vi "SLM_Control_Sample.vi"() -> ()   [LabVIEW 2016]
panel:
  in  "STOP button":bool
  out "Dffraction image":picture caption="Diffraction image"
  out "LG Beam image":picture
  out "Cylindrical lense image":picture caption="Cylindrical Lens image"
  out "Axicon image":picture
  out "Target image":picture
  out "Correction image":picture
  out "CGH image":picture caption="Tiled CGH image / Target image"
  out "Fresnel Lens image":picture
  out "2nd Display(LCOS) image":picture
  in  "?":T1(tab)
  in  "CGH  ON / OFF":bool=TRUE
  in  "LCOS type":string(combo)="X15223 series"
  in  "Corection image address":path
  in  "Target image address":path
  in  "Repetition Number":u32=100
  in  "Slip":i32
  in  "Cylindrical Lens":bool=TRUE
  in  "Cylindrical Focus/mm":i32=1000
  in  "WaveFront":bool=TRUE
  in  "Fresnel Lens":bool=TRUE
  in  "LUT":bool
  in  "2π Signal Level (0-255)":u8=210
  in  "Fresnel Focus/mm":i32=1000
  in  "Wave length/nm":u32=532
  out "Wave length/nm":u32=532
  in  "Mode Select":enum32{"Row", "Column"}(radio)
  in  "Rotation degree":dbl
  in  "Axicon Lens":bool=TRUE
  in  "Top level / πrad.":dbl=4.0
  in  "LG Beam":bool=TRUE
  in  "m":u32=1
  in  "p":u32=1
  in  "Diffraction":bool=TRUE
  in  "Mode Select2":enum32{"Row", "Column"}(radio)
  in  "gradation width":u32=1
  in  "gradation number":u32=2
  in  "Flip image":i32(listbox)
  in  "Beam size / mm":dbl
  in  "Additional phase mask (2πrad. at 0-255level) 2":path
  in  "Additional phase combination mode\nComplex amplitude / Amplitude 2":bool
  in  "Save 2nd Display image button":bool
  in  "Additional phase combination mode\nComplex amplitude / Amplitude 1":bool=TRUE
  in  "Monitor mumber":i32=2
  in  "Y PixelShift":i32
  in  "X PixelShift":i32
  in  "Additional phase mask (2πrad. at 0-255level) 1":path
  # "Sample code for\nLabVIEW"
  # "Basic Setting Parameter"
  # "LCOS-SLM"
  # "If a null address was input , all 0 pattern will appear."
  # "Target image"
  # "Corection"
  # "CGH"
  # "LCOS display settings"
  # "After press the STOP button, the BMP data save dialog will open."
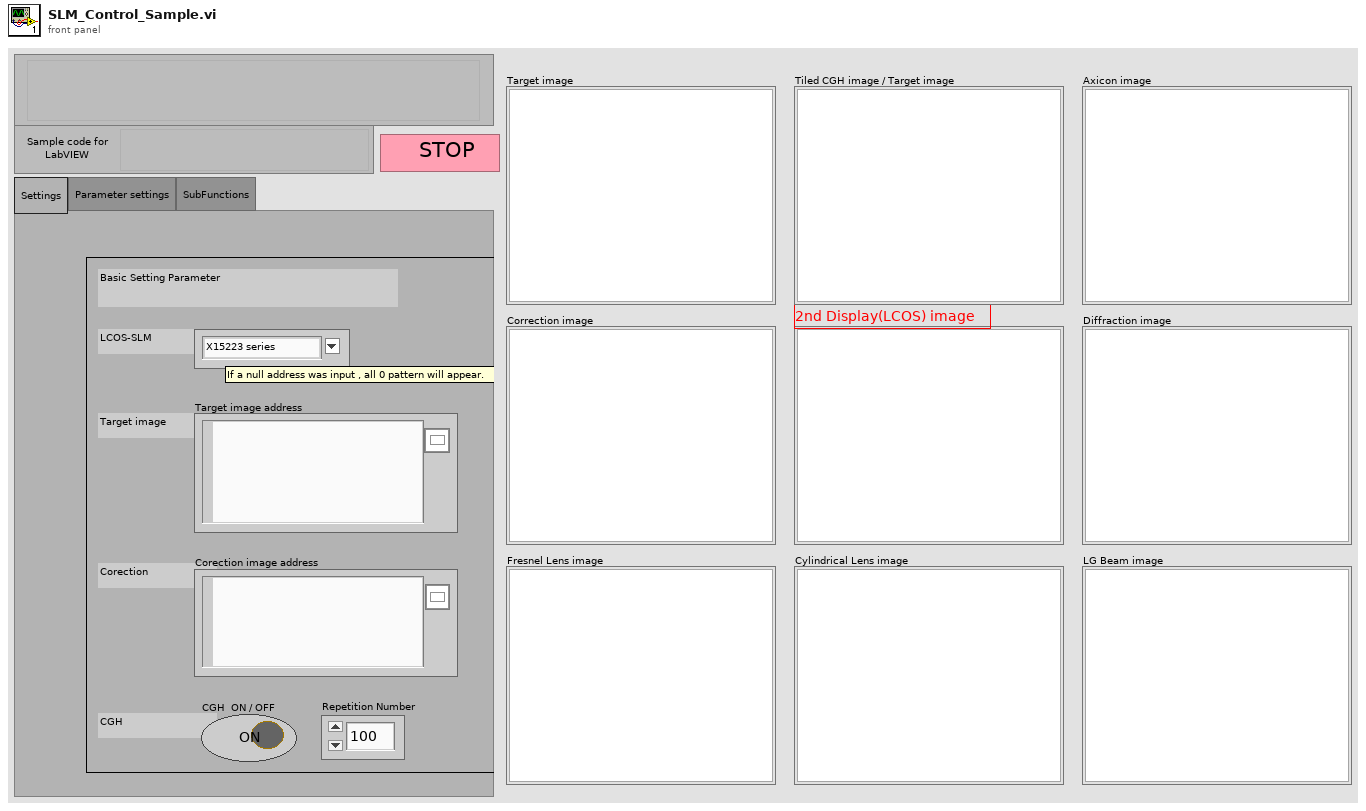
[diagram p1: front panel]
types:
  T1 = enum32{"Settings", "Parameter settings", "SubFunctions"}
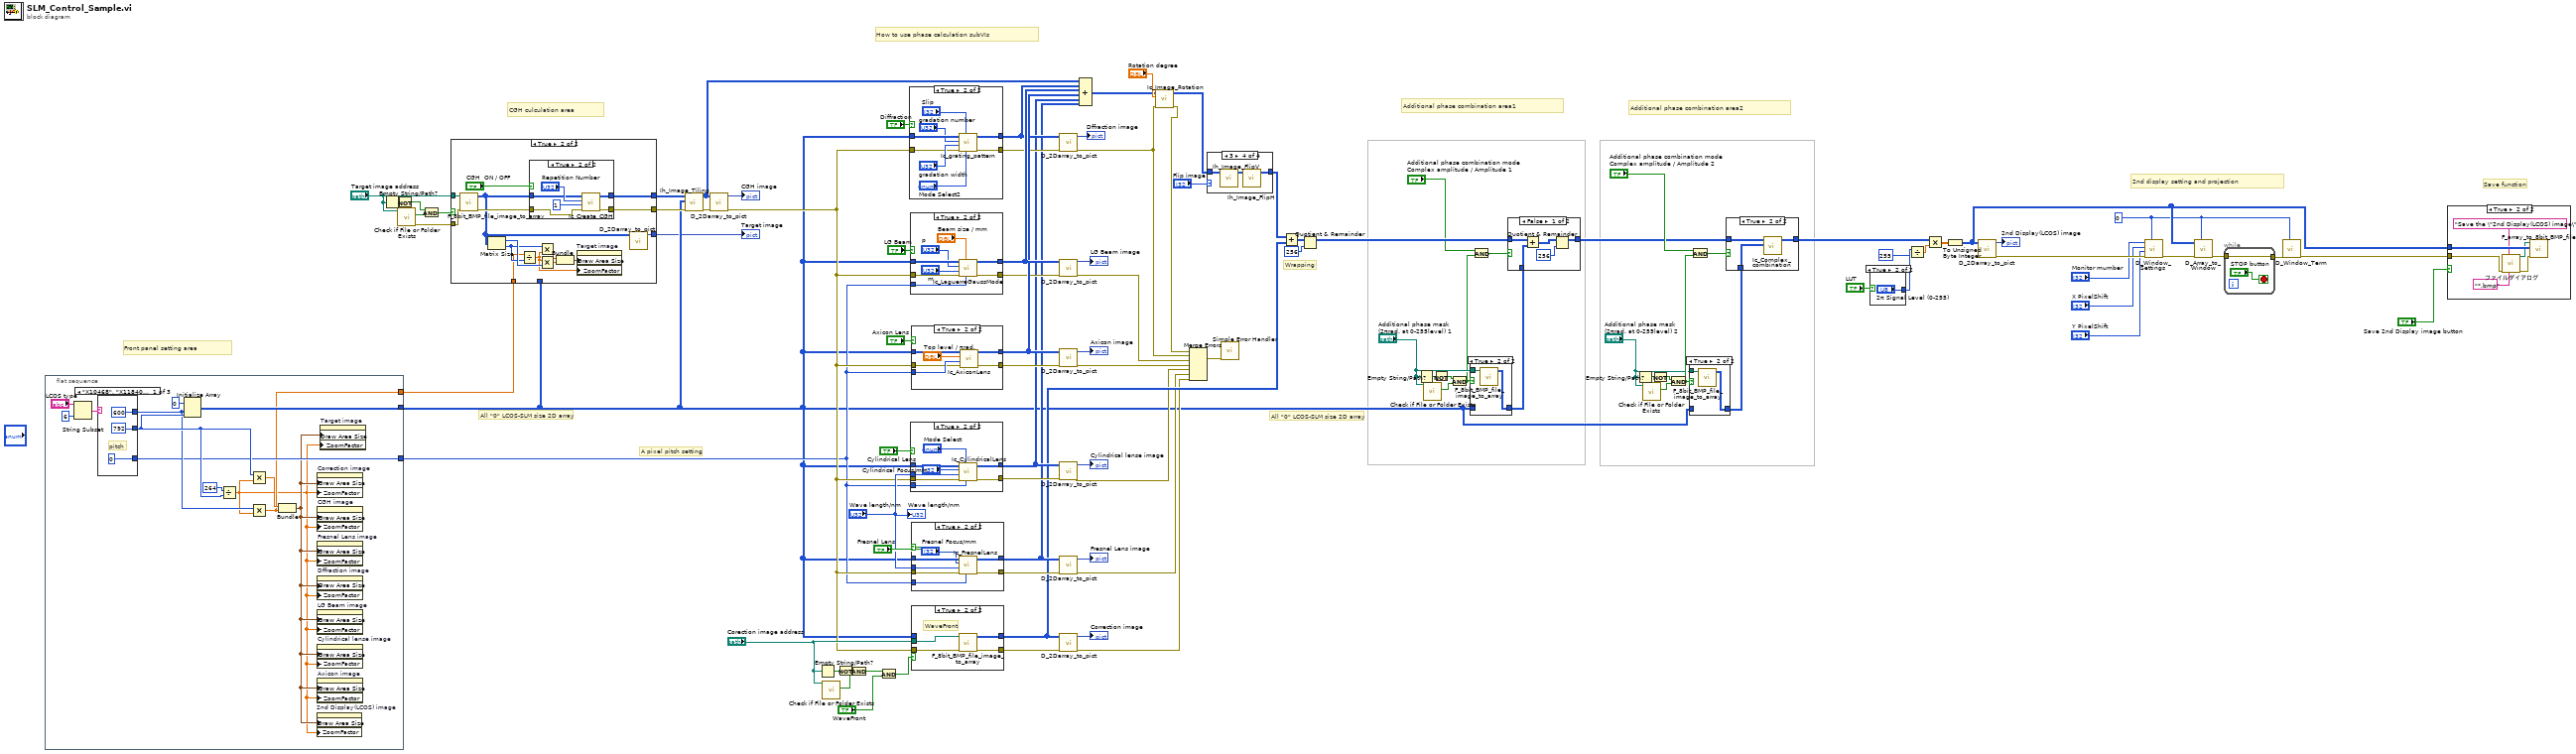
[diagram p0: block diagram]
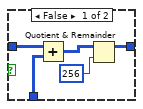
[diagram p3: hidden frame]
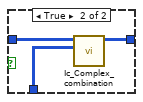
[diagram p5: hidden frame]
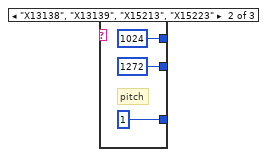
[diagram p7: hidden frame]
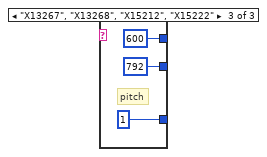
[diagram p8: hidden frame]
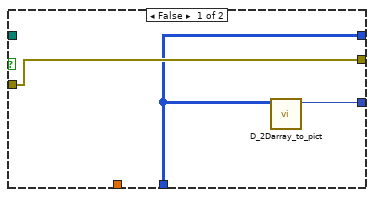
[diagram p9: hidden frame]
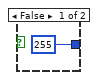
[diagram p16: hidden frame]
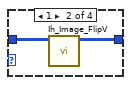
[diagram p18: hidden frame]
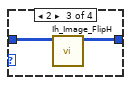
[diagram p19: hidden frame]
diagram:
  w16 = 0 ("Window Number (0...15)")
  # "All \"0\" LCOS-SLM size 2D array"
  # "Save function"
  # "All \"0\" LCOS-SLM size 2D array"
  # "A pixel pitch setting"
  # "How to use phase calculation subVIs"
  # "CGH culculation area"
  # "Front panel setting area"
  # "2nd display setting and projection"
  # "Additional phase combination area2"
  # "Additional phase combination area1"
  # "Wrapping"
  n1 = flat-sequence {
    tunnel: [w103] -> w3
    tunnel: [w102] -> w43
    tunnel: [w101] -> w2
    frame #0 {
      n2 = String Subset(string="LCOS type", length (rest)=6 ("長さ（残り）")) -> (substring=w108:string)  [unwired: 1 in]
      n3 = case shown="\"X10468\", \"X11840\", デフォルト" w108 {
        tunnel: [600 1024 600] -> w104
        tunnel: [792 1272 792] -> w105
        tunnel: [0 1 1] -> w102
        frame "X10468", "X11840", Default {
          # "pitch"
        }
        frame "X13138", "X13139", "X15213", "X15223" {
          # "pitch"
        }
        frame "X13267", "X13268", "X15212", "X15222" {
          # "pitch"
        }
      }
      n4 = Initialize Array(u8 0 ("要素"), w104, w105) -> (w103:u8[][])
      n5 = Divide(x=264, y=w105) -> (x/y=w99:dbl)
      n6 = Multiply(x=w105, y=w99) -> (x*y=w111:dbl)
      n7 = Multiply(x=w104, y=w99) -> (x*y=w101:dbl)
      n8 = Bundle(w111, w101) -> (w100:cluster{dbl, dbl})  [unwired: 1 in]
      n9 = property on="2nd Display(LCOS) image" class="Pict"("Draw Area Size"=w100, "ZoomFactor"=w99) -> ()  [unwired: 2 in, 2 out]
      n10 = property on="Correction image" class="Pict"("Draw Area Size"=w100, "ZoomFactor"=w99) -> ()  [unwired: 2 in, 2 out]
      n11 = property on="CGH image" class="Pict"("Draw Area Size"=w100, "ZoomFactor"=w99) -> ()  [unwired: 2 in, 2 out]
      n12 = property on="Fresnel Lens image" class="Pict"("Draw Area Size"=w100, "ZoomFactor"=w99) -> ()  [unwired: 2 in, 2 out]
      n13 = property on="Dffraction image" class="Pict"("Draw Area Size"=w100, "ZoomFactor"=w99) -> ()  [unwired: 2 in, 2 out]
      n14 = property on="LG Beam image" class="Pict"("Draw Area Size"=w100, "ZoomFactor"=w99) -> ()  [unwired: 2 in, 2 out]
      n15 = property on="Cylindrical lense image" class="Pict"("Draw Area Size"=w100, "ZoomFactor"=w99) -> ()  [unwired: 2 in, 2 out]
      n16 = property on="Axicon image" class="Pict"("Draw Area Size"=w100, "ZoomFactor"=w99) -> ()  [unwired: 2 in, 2 out]
      n17 = property on="Target image" class="Pict"("Draw Area Size"=w100, "ZoomFactor"=w99) -> ()  [unwired: 2 in, 2 out]
    }
  }
  n18 = Empty String/Path?(string/path="Target image address") -> (empty?=w74:bool)
  n19 = Not(x=w74) -> (.not. x?=w73:bool)
  n20 = call <vilib>:"Check if File or Folder Exists.vi"("path"="Target image address") -> ("error out"=w58:errorcluster, "file or folder exists?"=w71:bool)  [unwired: 8 in, 1 out]
  n21 = And(x=w73, y=w71) -> (x .and. y?=w72:bool)
  n22 = case shown="TRUE" w72 {
    tunnel: [w122 w137] -> w59
    tunnel: "Target image address" -> [_ w138]
    tunnel: w3 -> [w122 _]
    tunnel: w58 -> [w123 w135]
    tunnel: [w123 w133] -> w57
    tunnel: w2 -> [_ w126]
    tunnel: [w121 w125] -> w1
    frame False {
      n23 = call "D_2Darray_to_pict.vi"("2D array in"=w122) -> ("gray scale picture out"=w121:picture)  [unwired: 9 in, 1 out]
    }
    frame True {
      n24 = call "F_8bit_BMP_file_image_to_array.vi"("error in (no error)"=w135, "path to 8-bit BMP file"=w138) -> ("error out"=w134:errorcluster, "2D array out"=w124:u8[][])  [unwired: 8 in]
      n25 = Matrix Size(0:w124) -> (1:w131:i32, 2:w129:i32)
      n26 = Divide(x=w126, y=w129) -> (x/y=w127:dbl)
      n27 = case shown="TRUE" "CGH  ON / OFF" {
        tunnel: [w140 w145] -> w137
        tunnel: w124 -> [w140 w144]
        tunnel: w134 -> [w139 w142]
        tunnel: [w139 w141] -> w133
        frame False {
        }
        frame True {
          n28 = call "Ic_Create_CGH.vi"("2D array in"=w144, "Repetition Number"="Repetition Number", "progressBarOFF_0_ON_1"=u8 1, "error in (no error)"=w142) -> ("2D array out"=w145:u8[][], "error out"=w141:errorcluster)  [unwired: 5 in]
        }
      }
      n29 = Multiply(x=w129, y=w127) -> (x*y=w130:dbl)
      n30 = Multiply(x=w127, y=w131) -> (x*y=w132:dbl)
      n31 = Bundle(w130, w132) -> (w128:cluster{dbl, dbl})  [unwired: 1 in]
      n32 = property on="Target image" class="Pict"("Draw Area Size"=w128, "ZoomFactor"=w127) -> ()  [unwired: 2 in, 2 out]
      n33 = call "D_2Darray_to_pict.vi"("2D array in"=w124) -> ("gray scale picture out"=w125:picture)  [unwired: 9 in, 1 out]
    }
  }
  "Target image" <- w1
  n34 = call "Ih_Image_Tiling.vi"("error in (no error)"=w57, "2D array in (LCOS size buf)"=w3, "2D array in"=w59) -> ("error out"=w56:errorcluster, "2D array out"=w36:u8[][])  [unwired: 7 in]
  n35 = call "D_2Darray_to_pict.vi"("error in (no error)"=w56, "2D array in"=w36) -> ("error out"=w55:errorcluster, "gray scale picture out"=→"CGH image":picture)  [unwired: 8 in]
  n36 = Empty String/Path?(string/path="Corection image address") -> (empty?=w90:bool)
  n37 = call <vilib>:"Check if File or Folder Exists.vi"("path"="Corection image address") -> ("file or folder exists?"=w92:bool)  [unwired: 8 in, 2 out]
  n38 = Not(x=w90) -> (.not. x?=w91:bool)
  n39 = And(x=w91, y=w92) -> (x .and. y?=w87:bool)
  n40 = And(x=w87, y="WaveFront") -> (x .and. y?=w85:bool)
  n41 = case shown="TRUE" "Diffraction" {
    tunnel: w3 -> [w148 w156]
    tunnel: [w148 w152] -> w60
    tunnel: w55 -> [w147 w151]
    tunnel: [w147 w150] -> w51
    frame False {
    }
    frame True {
      n42 = call "Ic_grating_pattern.vi"("Row:0 or column:1"="Mode Select2", "Slip_factor"="Slip", "error in (no error)"=w151, "gradation width"="gradation width", "gradation number"="gradation number", "2D array in (LCOS size buf)"=w156) -> ("error out"=w150:errorcluster, "2D array out"=w152:u8[][])  [unwired: 4 in]
    }
  }
  n43 = case shown="TRUE" "LG Beam" {
    tunnel: w3 -> [w158 w166]
    tunnel: [w158 w165] -> w69
    tunnel: w43 -> [_ w162]
    tunnel: w55 -> [w157 w161]
    tunnel: [w157 w160] -> w50
    frame False {
    }
    frame True {
      n44 = call "Ic_LaguerreGaussMode.vi"("Pixel Pitch 0:20um_or_ 1:12.5um"=w162, "Beam size / mm"="Beam size / mm", "error in (no error)"=w161, "m :azimuthal index"="m", "p :radial index"="p", "2D array in (LCOS size buf)"=w166) -> ("error out"=w160:errorcluster, "2D array out"=w165:u8[][])  [unwired: 4 in]
    }
  }
  n45 = case shown="TRUE" "Cylindrical Lens" {
    tunnel: "Wave length/nm" -> [_ w174]
    tunnel: [w168 w176] -> w33
    tunnel: w3 -> [w168 w173]
    tunnel: w55 -> [w167 w172]
    tunnel: [w167 w171] -> w52
    tunnel: w43 -> [_ w169]
    frame False {
    }
    frame True {
      n46 = call "Ic_CylindricalLens.vi"("Pixel Pitch 0:20um_or_ 1:12.5um"=w169, "Mode Select"="Mode Select", "error in (no error)"=w172, "Wave Length / nm"=w174, "Cylindrical Focus / mm"="Cylindrical Focus/mm", "2D array in (LCOS size buf)"=w173) -> ("error out"=w171:errorcluster, "2D array out"=w176:u8[][])  [unwired: 4 in]
    }
  }
  n47 = case shown="TRUE" "Axicon Lens" {
    tunnel: w3 -> [w178 w184]
    tunnel: [w178 w183] -> w67
    tunnel: w43 -> [_ w181]
    tunnel: w55 -> [w177 w180]
    tunnel: [w177 w179] -> w49
    frame False {
    }
    frame True {
      n48 = call "Ic_AxiconLens.vi"("error in (no error)"=w180, "Pixel Pitch 0:20um_or_ 1:12.5um"=w181, "Top level / πrad."="Top level / πrad.", "2D array in (LCOS size buf)"=w184) -> ("error out"=w179:errorcluster, "2D array out"=w183:u8[][])  [unwired: 6 in]
    }
  }
  n49 = case shown="TRUE" "Fresnel Lens" {
    tunnel: "Wave length/nm" -> [_ w190]
    tunnel: w43 -> [_ w191]
    tunnel: w3 -> [w186 w193]
    tunnel: [w186 w192] -> w32
    tunnel: w55 -> [w185 w189]
    tunnel: [w185 w188] -> w53
    frame False {
    }
    frame True {
      n50 = call "Ic_FresnelLens.vi"("Pixel Pitch 0:20um_or_ 1:12.5um"=w191, "error in (no error)"=w189, "Wave length / nm"=w190, "Focus / mm"="Fresnel Focus/mm", "2D array in (LCOS size buf)"=w193) -> ("error out"=w188:errorcluster, "2D array out"=w192:u8[][])  [unwired: 5 in]
    }
  }
  n51 = case shown="TRUE" w85 {
    tunnel: "Corection image address" -> [_ w198]
    tunnel: [w195 w199] -> w31
    tunnel: w3 -> [w195 _]
    tunnel: w55 -> [w194 w197]
    tunnel: [w194 w196] -> w54
    frame False {
    }
    frame True {
      # "WaveFront"
      n52 = call "F_8bit_BMP_file_image_to_array.vi"("error in (no error)"=w197, "path to 8-bit BMP file"=w198) -> ("error out"=w196:errorcluster, "2D array out"=w199:u8[][])  [unwired: 8 in]
    }
  }
  n53 = call "D_2Darray_to_pict.vi"("error in (no error)"=w51, "2D array in"=w60) -> ("error out"=w46:errorcluster, "gray scale picture out"=→"Dffraction image":picture)  [unwired: 8 in]
  n54 = call "D_2Darray_to_pict.vi"("error in (no error)"=w50, "2D array in"=w69) -> ("error out"=w47:errorcluster, "gray scale picture out"=→"LG Beam image":picture)  [unwired: 8 in]
  n55 = call "D_2Darray_to_pict.vi"("error in (no error)"=w49, "2D array in"=w67) -> ("error out"=w48:errorcluster, "gray scale picture out"=→"Axicon image":picture)  [unwired: 8 in]
  n56 = call "D_2Darray_to_pict.vi"("error in (no error)"=w52, "2D array in"=w33) -> ("error out"=w30:errorcluster, "gray scale picture out"=→"Cylindrical lense image":picture)  [unwired: 8 in]
  n57 = call "D_2Darray_to_pict.vi"("error in (no error)"=w53, "2D array in"=w32) -> ("error out"=w29:errorcluster, "gray scale picture out"=→"Fresnel Lens image":picture)  [unwired: 8 in]
  n58 = call "D_2Darray_to_pict.vi"("error in (no error)"=w54, "2D array in"=w31) -> ("error out"=w28:errorcluster, "gray scale picture out"=→"Correction image":picture)  [unwired: 8 in]
  n59 = Compound Arithmetic op=ADD(w36, w60, w69, w67, w33, w32) -> (w77:u8[][])
  n60 = call "Ic_Image_Rotation.vi"("error in (no error)"=w46, "degree"="Rotation degree", "2D array in"=w77) -> ("error out"=w45:errorcluster, "2D array out"=w82:u8[][])  [unwired: 7 in]
  n61 = Merge Errors(w45, w46, w47, w48, w30, w29, w28) -> (w44:errorcluster)
  n62 = case shown="3" "Flip image" {
    tunnel: w82 -> [w200 w202 w204 w205]
    tunnel: [w200 w201 w203 w206] -> w76
    frame 0, Default {
    }
    frame 1 {
      n63 = call "Ih_Image_FlipV.vi"("2D array in"=w202) -> ("Flip V 2D array out"=w201:u32[][])  [unwired: 10 in]
    }
    frame 2 {
      n64 = call "Ih_Image_FlipH.vi"("2D array in"=w204) -> ("Flip H 2D array out"=w203:u32[][])  [unwired: 10 in]
    }
    frame 3 {
      n65 = call "Ih_Image_FlipV.vi"("2D array in"=w205) -> ("Flip V 2D array out"=w207:u32[][])  [unwired: 10 in]
      n66 = call "Ih_Image_FlipH.vi"("2D array in"=w207) -> ("Flip H 2D array out"=w206:u32[][])  [unwired: 10 in]
    }
  }
  n67 = call <vilib>:"Simple Error Handler.vi"("error in (no error)"=w44) -> ()  [unwired: 4 in, 5 out]
  n68 = Add(x=w76, y=w31) -> (x+y=w35:u32[][])
  n69 = Quotient & Remainder(x=w35, y=256) -> (x-y*floor(x/y)=w27:u32[][])  [unwired: 1 out]
  n70 = Empty String/Path?(string/path="Additional phase mask (2πrad. at 0-255level) 1") -> (empty?=w21:bool)
  n71 = call <vilib>:"Check if File or Folder Exists.vi"("path"="Additional phase mask (2πrad. at 0-255level) 1") -> ("file or folder exists?"=w25:bool)  [unwired: 8 in, 2 out]
  n72 = Not(x=w21) -> (.not. x?=w24:bool)
  n73 = And(x=w24, y=w25) -> (x .and. y?=w19:bool)
  n74 = case shown="TRUE" w19 {
    tunnel: "Additional phase mask (2πrad. at 0-255level) 1" -> [_ w210]
    tunnel: w3 -> [w208 _]
    tunnel: [w208 w209] -> w22
    frame False {
    }
    frame True {
      n75 = call "F_8bit_BMP_file_image_to_array.vi"("path to 8-bit BMP file"=w210) -> ("2D array out"=w209:u8[][])  [unwired: 9 in, 1 out]
    }
  }
  n76 = And(x="Additional phase combination mode\nComplex amplitude / Amplitude 1", y=w19) -> (x .and. y?=w18:bool)
  n77 = case shown="FALSE" w18 {
    tunnel: w27 -> [w215 w218]
    tunnel: [w211 w216] -> w6
    tunnel: w22 -> [w214 w217]
    frame False {
      n78 = Add(x=w215, y=w214) -> (x+y=w212:u32[][])
      n79 = Quotient & Remainder(x=w212, y=256) -> (x-y*floor(x/y)=w211:u32[][])  [unwired: 1 out]
    }
    frame True {
      n80 = call "Ic_Complex_combination.vi"("2D array in 2"=w217, "2D array in"=w218) -> ("2D array out"=w216:u8[][])  [unwired: 9 in]
    }
  }
  n81 = Empty String/Path?(string/path="Additional phase mask (2πrad. at 0-255level) 2") -> (empty?=w12:bool)
  n82 = call <vilib>:"Check if File or Folder Exists.vi"("path"="Additional phase mask (2πrad. at 0-255level) 2") -> ("file or folder exists?"=w15:bool)  [unwired: 8 in, 2 out]
  n83 = Not(x=w12) -> (.not. x?=w14:bool)
  n84 = And(x=w14, y=w15) -> (x .and. y?=w11:bool)
  n85 = case shown="TRUE" w11 {
    tunnel: "Additional phase mask (2πrad. at 0-255level) 2" -> [_ w221]
    tunnel: w3 -> [w219 _]
    tunnel: [w219 w220] -> w13
    frame False {
    }
    frame True {
      n86 = call "F_8bit_BMP_file_image_to_array.vi"("path to 8-bit BMP file"=w221) -> ("2D array out"=w220:u8[][])  [unwired: 9 in, 1 out]
    }
  }
  n87 = And(x="Additional phase combination mode\nComplex amplitude / Amplitude 2", y=w11) -> (x .and. y?=w10:bool)
  n88 = case shown="TRUE" w10 {
    tunnel: w6 -> [w226 w229]
    tunnel: [w222 w227] -> w7
    tunnel: w13 -> [w225 w228]
    frame False {
      n89 = Add(x=w226, y=w225) -> (x+y=w223:u32[][])
      n90 = Quotient & Remainder(x=w223, y=256) -> (x-y*floor(x/y)=w222:u32[][])  [unwired: 1 out]
    }
    frame True {
      n91 = call "Ic_Complex_combination.vi"("2D array in 2"=w228, "2D array in"=w229) -> ("2D array out"=w227:u8[][])  [unwired: 9 in]
    }
  }
  n92 = case shown="TRUE" "LUT" {
    tunnel: [255 ("2π Signal Level (0-255)") "2π Signal Level (0-255)"] -> w95
    frame False {
    }
    frame True {
    }
  }
  n93 = Divide(x=w95, y=255) -> (x/y=w96:dbl)
  n94 = Multiply(x=w7, y=w96) -> (x*y=w94:dbl[][])
  n95 = To Unsigned Byte Integer(number=w94) -> (unsigned 8bit integer=w40:u8[][])
  n96 = call "D_2Darray_to_pict.vi"("2D array in"=w40) -> ("error out"=w42:errorcluster, "gray scale picture out"=→"2nd Display(LCOS) image":picture)  [unwired: 9 in]
  n97 = call "D_Window_Settings.vi"("Window Number (0...15)"=w16, "error in (no error)"=w42, "YPixelShift"="Y PixelShift", "XPixelShift"="X PixelShift", "Monitor mumber"="Monitor mumber") -> ("error out"=w41:errorcluster)  [unwired: 6 in]
  n98 = call "D_Array_to_Window.vi"("Window Number (0...15)"=w16, "error in (no error)"=w41, "Image Pixels (U8)"=w40) -> ("error out"=w5:errorcluster)  [unwired: 8 in]
  n99 = while {
    tunnel: w5 -> [w233]
    tunnel: [w233] -> w4
    stop <- "STOP button" stop-if-true
  }
  n100 = call "D_Window_Term.vi"("Window Number (0...15)"=w16, "error in (no error)"=w4) -> ("error out"=w17:errorcluster)  [unwired: 9 in]
  n101 = case shown="TRUE" "Save 2nd Display image button" {
    tunnel: w17 -> [_ w235]
    tunnel: w40 -> [_ w239]
    frame False {
    }
    frame True {
      n102 = call "ファイルダイアログ"("prompt"="Save the \"2nd Display(LCOS) image\"", "error in"=w235, "pattern (all files)"="*.bmp") -> ("selected path"=w238:path, "error out"=w234:errorcluster)  [unwired: 9 in, 2 out]
      n103 = call "F_array_to_8bit_BMP_file.vi"("error in (no error)"=w234, "2D array in"=w239, "path to save BMP file"=w238) -> ()  [unwired: 8 in, 1 out]
    }
  }
  "Wave length/nm" <- "Wave length/nm"
